vi "UpdateYear.vi"(6 "Status ref":refnum<vi>, 8 "error in":errorcluster, 11 "Year Folder":path) -> (0 "error out":errorcluster, 3 "Comics":T1[](array[typedef]) {"Cover Price" format="$%.2g"})   [LabVIEW 2022 SP3]
uses:
  TypeDefs/Comic.ctl
  TypeDefs/Character.ctl
  TypeDefs/Creator.ctl
  TypeDefs/Variant.ctl
  14f7bc4a-da15-464d-b3b9-b5eb56e3d304.vi
  <vilib>/Comparison/Less/Less Functor/Less Functor.lvclass
panel:
  out "Current Week":string
  out "Current Comic":string
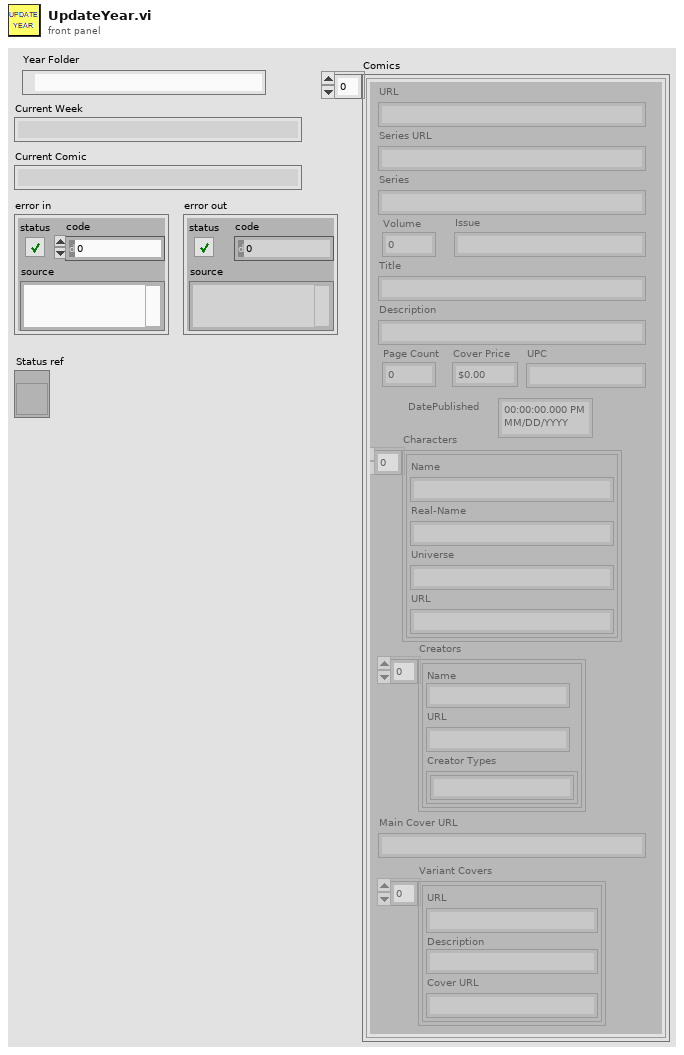
[diagram p1: front panel]
types:
  T1 = typedef "Comic.ctl" = cluster{"URL":string, "Series URL":string, "Series":string, "Volume":i32, "Issue":string, "Title":string, "Description":string, "Page Count":i32, "Cover Price":dbl, "UPC":string, "Characters":T2[], "Creators":T3[], "Main Cover URL":string, "Variant Covers":T4[], "DatePublished":timestamp}
  T2 = typedef "Character.ctl" = cluster{"Name":string, "Real-Name":string, "Universe":string, "URL":string}
  T3 = typedef "Creator.ctl" = cluster{"Name":string, "URL":string, "Creator Types":string[]}
  T4 = typedef "Variant.ctl" = cluster{"URL":string, "Description":string, "Cover URL":string}
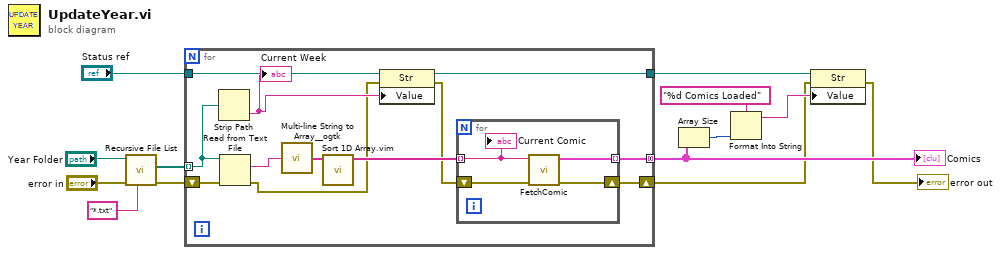
[diagram p0: block diagram]
diagram:
  n1 = call <vilib>:"Recursive File List.vi"("pattern"="*.txt", "error in (no error)"="error in", "Folder Path"="Year Folder") -> ("error out"=w10:errorcluster, "All Files in Dir"=w9:path[])  [unwired: 4 in, 3 out]
  n2 = for {
    tunnel: [w23] -> w6 mode=concatenating
    shift-right: [w21] -> w2
    shift-left: w10 -> [w20]
    tunnel: w9 -> [w19] mode=indexing
    tunnel: "Status ref" -> [w18]
    tunnel: [w16] -> w7
    n3 = Strip Path(path=w19) -> (name=w17:string)  [unwired: 1 out]
    "Current Week" <- w17
    n4 = Read from Text File(file (use dialog)=w19, error in=w20) -> (text=w25:string, error out=w15:errorcluster)  [unwired: 2 in, 2 out]
    n5 = call <userlib>:"Multi-line String to Array__ogtk.vi"("string"=w25) -> ("lines"=w24:string[])
    n6 = call "Sort 1D Array.vim"("unsorted array"=w24) -> ("sorted array"=w22:string[])  [unwired: 10 in]
    n7 = property class="Str"(reference=w18, error in=w15, "Value"=w17) -> (reference out=w16:refnum<vi>, error out=w14:errorcluster)
    n8 = for {
      tunnel: w22 -> [w29] mode=indexing
      shift-right: [w27] -> w21
      shift-left: w14 -> [w28]
      tunnel: [w26] -> w23 mode=indexing
      n9 = call "FetchComic.vi"("error in (no error)"=w28, "ComicURL"=w29) -> ("error out"=w27:errorcluster, "Comic"=w26:T1)  [unwired: 8 in]
      "Current Comic" <- w29
    }
  }
  "Comics" <- w6
  n10 = Array Size(array=w6) -> (size(s)=w5:i32)
  n11 = Format Into String(format string="%d Comics Loaded", w5) -> (resulting string=w3:string)  [unwired: 2 in, 1 out]
  n12 = property class="Str"(reference=w7, error in=w2, "Value"=w3) -> (error out=→"error out":errorcluster)  [unwired: 1 out]
